vi "DAQmx Write (Digital 1D Wfm NChan 1Samp).vi"(0 "task/channels in":refnum<k21>, 1 "auto start":bool=TRUE, 7 "data":digitalwaveform[](array[waveform]), 9 "timeout":dbl=10.0 format="%0.2f", 11 "error in":errorcluster) -> (4 "task out":refnum<k21>, 10 "number of samples written per channel":u32, 15 "error out":errorcluster)   [LabVIEW 2018]
doc: "Writes a digital waveform that contains a single sample to each channel in a task that contains one or more digital output channels."
uses:
  nilvaiu.dll
panel:
  # "sample #"
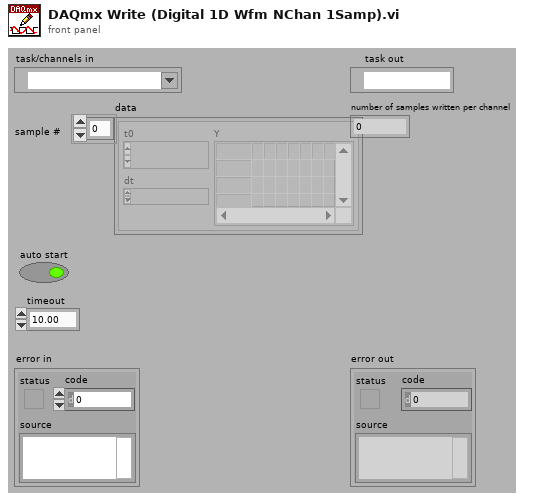
[diagram p1: front panel]
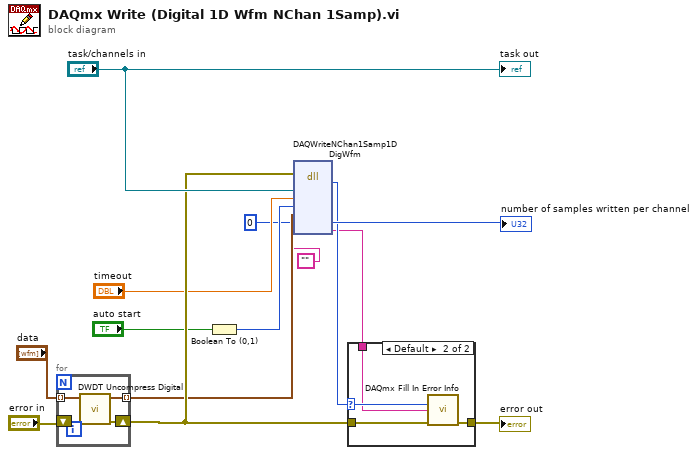
[diagram p0: block diagram]
diagram:
  n1 = for {
    tunnel: "data" -> [w18] mode=indexing
    tunnel: [w17] -> w9 mode=indexing
    shift-right: [w16] -> w10
    shift-left: "error in" -> [w15]
    n2 = call "DWDT Uncompress Digital.vi"("error in (no error)"=w15, "compressed digital waveform"=w18) -> ("error out"=w16:errorcluster, "uncompressed digital waveform"=w17:digitalwaveform)  [unwired: 8 out]
  }
  n3 = Boolean To (0,1)(Boolean="auto start") -> (0, 1=w4:i16)
  n4 = dll-call lib="nilvaiu.*" fn="DAQWriteNChan1Samp1DDigWfm"(error in=w10, "taskID"="task/channels in", "timeout"="timeout", "autoStart"=w4, "data"=w9, "numSamplesWriten"=u32 0, "extendedErrorInfo"="") -> (w5:i32, "numSamplesWriten"=→"number of samples written per channel":u32, "extendedErrorInfo"=w3:string)  [unwired: 4 in, 4 out]
  n5 = case shown="Default" w5 {
    selector: w5 -> [_ w21]
    tunnel: w10 -> [w19 w23]
    tunnel: [w19 w22] -> w13
    tunnel: w3 -> [_ w20]
    frame 0 {
    }
    frame Default {
      n6 = call "DAQmx Fill In Error Info.vi"("status code"=w21, "extended error info"=w20, "error in"=w23) -> ("error out"=w22:errorcluster)  [unwired: 1 in, 11 out]
    }
  }
  "error out" <- w13
  "task out" <- "task/channels in"
